vi "Convert NI Time Stamp to AIM Time Stamp.vi"(11 "Time Stamp":timestamp format="%<%.6X\n%x>T") -> (3 "IRIG Time Stamp":T1={"Days of year"=1, "Hours"=0, "Minutes"=0, "Seconds"=0, "Milliseconds"=0})   [LabVIEW 2020]
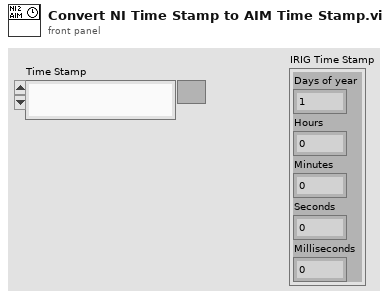
[diagram p1: front panel]
types:
  T1 = cluster{"Days of year":u32, "Hours":u32, "Minutes":u32, "Seconds":u32, "Milliseconds":u32}
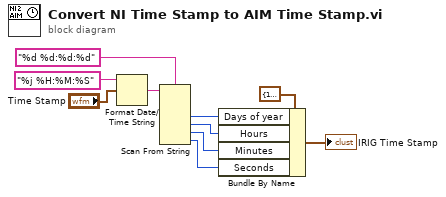
[diagram p0: block diagram]
diagram:
  n1 = Format Date/Time String(time format string (%c)="%j %H:%M:%S" ("format string"), seconds (now)="Time Stamp") -> (date/time string=w6:string)  [unwired: 1 in]
  n2 = Scan From String(format string="%d %d:%d:%d", input string=w6) -> (output 1=w5:i32, output 2=w4:i32, output 3=w3:i32, output 4=w2:i32)  [unwired: 6 in, 3 out]
  n3 = Bundle By Name(cluster=T1 {"Days of year"=1, "Hours"=0, "Minutes"=0, "Seconds"=0, "Milliseconds"=0} ("IRIG Time Stamp"), "Days of year"=w5, "Hours"=w4, "Minutes"=w3, "Seconds"=w2) -> (→"IRIG Time Stamp":T1)
